vi "MU Calibration adjust Analog By Analyze Result.vi"(8 "error in (no error)":errorcluster, 10 "analyzeResult":T1, 11 "calibration":T2) -> (0 "error out":errorcluster, 3 "function return":bool)   [LabVIEW 2017, in "MU_3SL_interface.lvlib"]
doc: "MU_PUBLIC bool MU_Calibration_adjustAnalogByAnalyzeResult(\n MU_Calibration* calibration,\n const MU_CalibrationAnalyzeResult* analyzeResult);"
uses:
  MU_3SL_interface.lvlib
  handles/CalibrationHandle.ctl
  handles/CalibrationAnalyzeResultHandle.ctl
  lib/MU_3SL_interface.dll
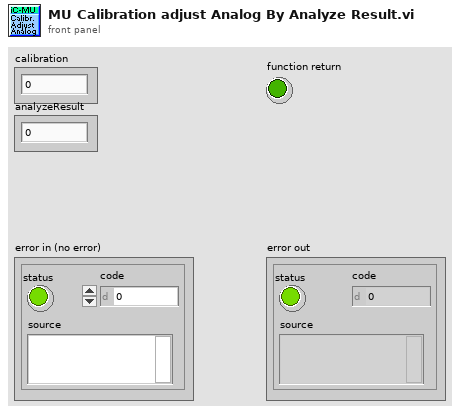
[diagram p1: front panel]
types:
  T1 = typedef "MU_3SL_interface.lvlib/CalibrationAnalyzeResultHandle.ctl" = u64
  T2 = typedef "MU_3SL_interface.lvlib/CalibrationHandle.ctl" = u64
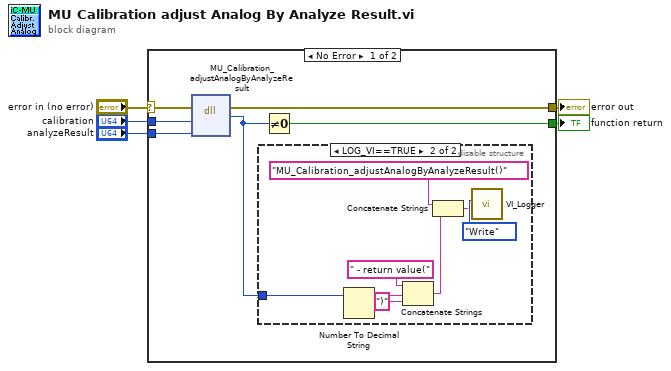
[diagram p0: block diagram]
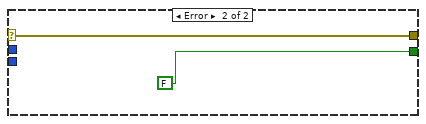
[diagram p3: hidden frame]
diagram:
  n1 = case shown="No Error" "error in (no error)" {
    selector: "error in (no error)" -> [w8 w21]
    tunnel: [w11 FALSE] -> w5
    tunnel: [w7 w21] -> w4
    tunnel: "calibration" -> [w10 _]
    tunnel: "analyzeResult" -> [w9 _]
    frame No Error {
      n2 = dll-call lib="C:/Users/bes/AppData/Roaming/work/mu_9so/icsubmodules/soft_mu_3sl_master/lv_interface/lib/MU_3SL_interface**.*" fn="MU_Calibration_adjustAnalogByAnalyzeResult"(error in=w8, "calibration"=w10, "analyzeResult"=w9) -> (error out=w7:errorcluster, "return type"=w6:u8)  [unwired: 4 in, 1 out]
      n3 = disable-structure shown="LOG_VI==TRUE" {
        disable-tunnel: w6 -> [_ w17]
        frame condition #0 {
        }
        frame condition #1 (active) {
          n4 = Number To Decimal String(number=w17) -> (decimal integer string=w16:string)  [unwired: 1 in]
          n5 = Concatenate Strings(" - return value(" ("string"), w16, ")" ("string")) -> (w15:string)
          n6 = Concatenate Strings("MU_Calibration_adjustAnalogByAnalyzeResult()" ("Info in"), w15) -> (w14:string)
          n7 = call "VI_Logger.vi"("Action (Read)"=enum16{"Write", "Read"}."Write", "Info in"=w14) -> ()  [unwired: 8 in, 2 out]
        }
      }
      n8 = Not Equal To 0?(x=w6) -> (x != 0?=w11:bool)
    }
    frame Error {
    }
  }
  "function return" <- w5
  "error out" <- w4
